vi "play_FXP_AFMss_MPC_DistEst_singleAxis.vi"() -> ()   [LabVIEW 2017]
uses:
  fpga_VIs/fixed-point/single-axis/fxp_mpc/fgm_pipiline/quadProgParams_pipe.ctl
  fpga_VIs/fixed-point/typeDefs/FXPControlParams_distEst.ctl
  <vilib>/Analysis/Matrix/Datatypes/RealMatrix.ctl
  fpga_fp_interface_lib/fpga_interface_types/boolean_indicators.ctl
  controls/ObserverMatrices.ctl
  <vilib>/userdefined/High Color/nirio_resource_hc.ctl
  <vilib>/Utility/error.llb/DialogType.ctl
  <vilib>/Utility/file.llb/Read Delimited Spreadsheet (DBL).vi
  <vilib>/FPGAPlugInAG/cRIO-9082/niLvFpga_Open_cRIO-9082.vi
  <vilib>/rvi/interface/common/dynamic/niFpgaDynamicAddResources.vi
  <vilib>/FPGAPlugInAG/Dynamic/niLvFpga_Reset_Dynamic.vi
  <vilib>/rvi/interface/common/niFpgaWaitOnOcc.vi
  <vilib>/Utility/error.llb/Error Cluster From Error Code.vi
  <vilib>/rvi/errors/niLvFpgaAdjustHostInterfaceError.vi
  <vilib>/FPGAPlugInAG/Dynamic/niLvFpga_Run_Dynamic.vi
  <vilib>/RVI Host/nirviSupport.llb/nirviErrorClusterFromErrorCode.vi
  fpga_fp_interface_lib/write_FP_data_to_fpga.vi
  fpga_fp_interface_lib/acquire_FXP_18-5_FIFO_1.vi
  <vilib>/Analysis/Matrix/Numeric/Conversions/Array To Matrix - RA2.vi
  <vilib>/Utility/file.llb/Write To Spreadsheet File (DBL).vi
  <vilib>/FPGAPlugInAG/Dynamic/niLvFpga_Close_Dynamic.vi
  <vilib>/rvi/interface/nirviOpenFPGA/nirviOpenFPGA.xnode
  FPGA Bitfiles/XYpeizocontrol_FPGATarget_FXPAFMssMPCsingle_axis.lvbitx
  <vilib>/rvi/interface/nirviMethod/nirviMethod.xnode
  <vilib>/rvi/interface/nirviReadWriteControl/nirviReadWriteControl.xnode
  <vilib>/rvi/interface/nirviCloseFPGA/nirviCloseFPGA.xnode
  <vilib>/rvi/errors/niLvFpgaMergeErrorWithErrorCode.vi
  <vilib>/rvi/interface/Simulation/niFpgaSimulationCallBeginRW.vi
  <vilib>/rvi/interface/nirviMethod/StockFPGA_InlinedMethodWaitForSingleIRQ.vi
  <vilib>/FPGAPlugInAG/Dynamic/niLvFpga_WaitOnIrq_Dynamic.vi
  <vilib>/FPGAPlugInAG/Dynamic/niLvFpga_AcknowledgeIrq_Dynamic.vi
  <vilib>/FPGAPlugInAG/Dynamic/niLvFpga_ConfigureFifo_Dynamic.vi
  NiFpgaLv.dll
  <vilib>/Analysis/Matrix/NI_Matrix.lvlib
  <vilib>/FPGAPlugInAG/Dynamic/niLvFpga_WriteFifo_Dynamic.vi
  labview/utils_lib/utils.lvlib
panel:
  out "first row":dbl[](array[numeric])
  out "elements left":i32=1
  in  "N_sat":i32
  in  "wsat_s":T1
  in  "d_s":T1
  in  "N_hyst":i32
  in  "w-s":T1
  in  "r_s":T1
  in  "TF Order":i32
  in  "den":T1
  in  "num":T1
  out "u_k out":fxp<+/-,32,5>
  out "size(s)":i32[](array[numeric])
  in  "Tab Control":T2(tab)
  in  "traj_path":path=path "C:/Users/arnold/Documents/MATLAB/afm_mpc_journal/data/MPCControls01.csv"
  in  "control_data_path":path=path "C:/Users/arnold/Documents/MATLAB/afm_mpc_journal/data/MPCControls01.csv"
  in  "outputDataPath":path=path "Z:/mpc-journal/step-exps/expOut_multiAxis_mpc_tmp.csv"
  in  "dry_run":bool
  out "XY Graph":cluster{dbl[], "2D Data Out":dbl[]}[](graph)
  out "QP_params":T3={"maxIter"=0, "nuN"=24, "Ns_mpc"=0, "-beta"=-0.9987945556640625, "beta+1"=1.9987945556640625}
  out "ControlParams":T4={"umax"=3.0, "Ns_obs/cntrl"=0, "ref_f_VEC"=[0.0, 0.0], "du_max"=0.0}
  in  "TsTicks":i32=1600
  in  "umax":dbl=1.0 format="%#_13g"
  in  "ymax":dbl=4.0 format="%#_13g"
  in  "Iters":i32=25
  in  "SettleTicks":i32=10
  in  "ABORT":bool
  out "Fifo matrix TimeOUt":bool
  in  "ref":dbl=1.0 format="%#_13g"
  out "Loop Ticks (benchmark)":i16
  in  "maxIter":u16=20
  out "boolean  indicators":T5
  out "error out (stage 2)":errorcluster
  out "Error Out (stage 1)":errorcluster
  out "x-x(0)":fxp<+/-,18,5>
  out "ControlMatrices":T6
  out "MPC matrices":dbl[][](array[numeric])
  out "result_data":T1
  out "Empty Elements Remaining":u32
  # "NOTE: Ns is the number of states in the plant. The number of states in the \nobserver is Ns+1. Thus, for B, L, C, and A, we use NS+1. For K and Xss, we use Ns\nbecause the controller does not operate on the disturbance state, Xd."
  # "yk\nulin\ndu\nu_inv\nIpow\nX"
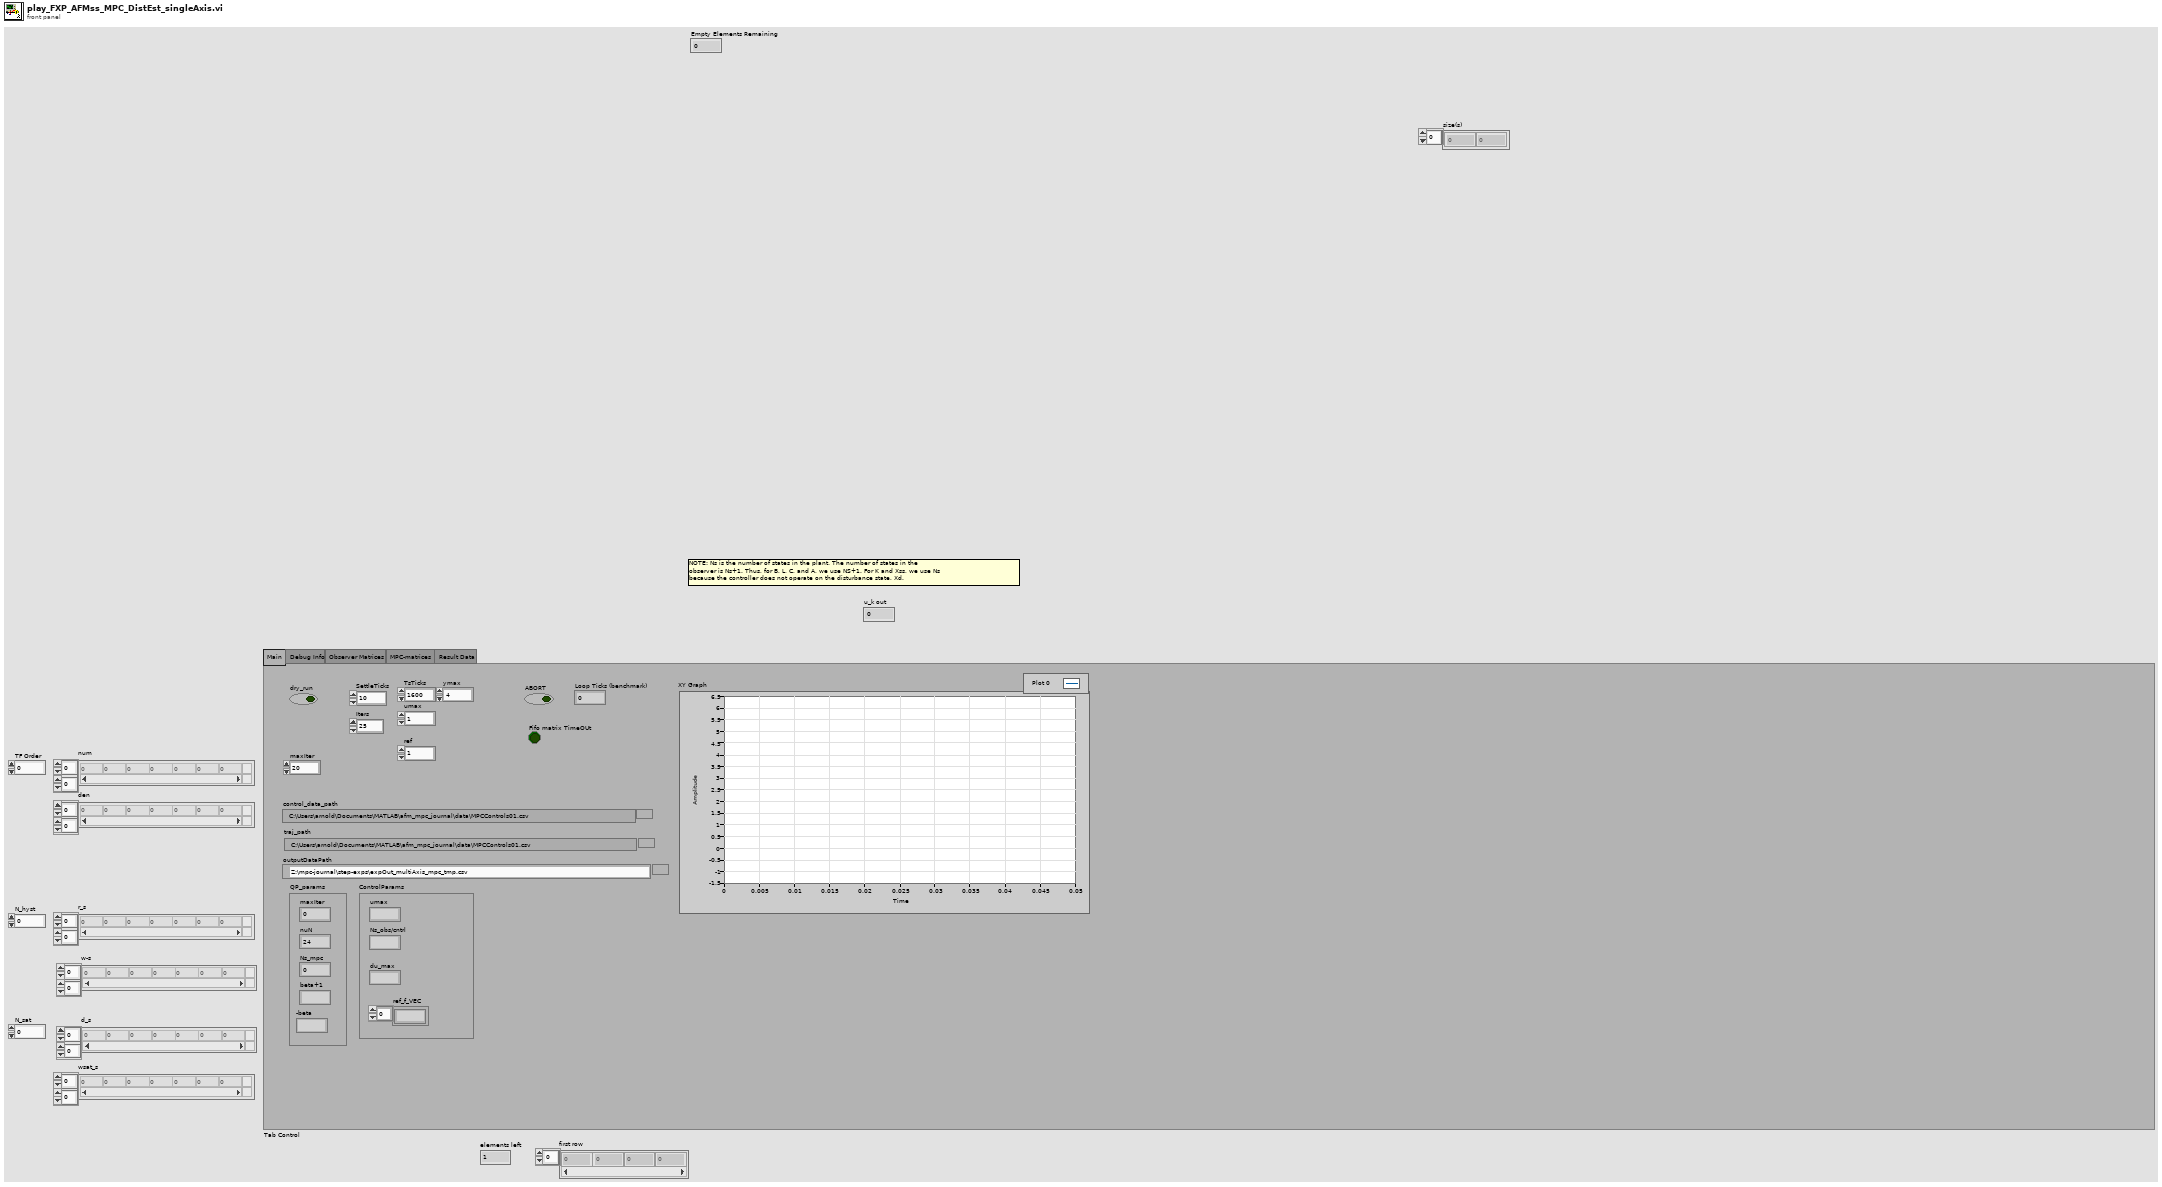
[diagram p1: front panel]
types:
  T1 = typedef "NI_Matrix.lvlib/RealMatrix.ctl" = dbl[][]
  T2 = enum32{"Main", "Debug Info", "Observer Matrices", "MPC-matrices", "Result Data"}
  T3 = typedef "quadProgParams_pipe.ctl" = cluster{"maxIter":u16, "nuN":u16, "Ns_mpc":u16, "-beta":fxp<+/-,18,2>, "beta+1":fxp<+/-,18,2>}
  T4 = typedef "FXPControlParams_distEst.ctl" = cluster{"umax":fxp<+/-,18,5>, "Ns_obs/cntrl":u8, "ref_f_VEC":fxp<+/-,32,5>[], "du_max":fxp<+/-,18,5>}
  T5 = typedef "boolean_indicators.ctl" = cluster{"unstable-z-traj":bool, "input fifo time-out":bool, "logging fifo timeout":bool, "scanning finished":bool, "unstable-x-traj":bool, "unstable-y-traj":bool, "ABORT":bool, "All Measurements Done":bool, "fpga_finished":bool}
  T6 = typedef "ObserverMatrices.ctl" = cluster{"Az":fxp<+/-,32,4>[][], "Bz":dbl[][], "Lz":dbl[][], "Kz":dbl[][], "NxNu":dbl[][]}
  T7 = typedef "nirio_resource_hc.ctl" = tag
  T8 = cluster{"unstable-z-traj":bool, "input fifo time-out":bool, "logging fifo timeout":bool, "scanning finished":bool, "unstable-x-traj":bool, "unstable-y-traj":bool, "ABORT":bool, "All Measurements Done":bool, "fpga_finished":bool}
  T9 = typedef "DialogType.ctl" = u16
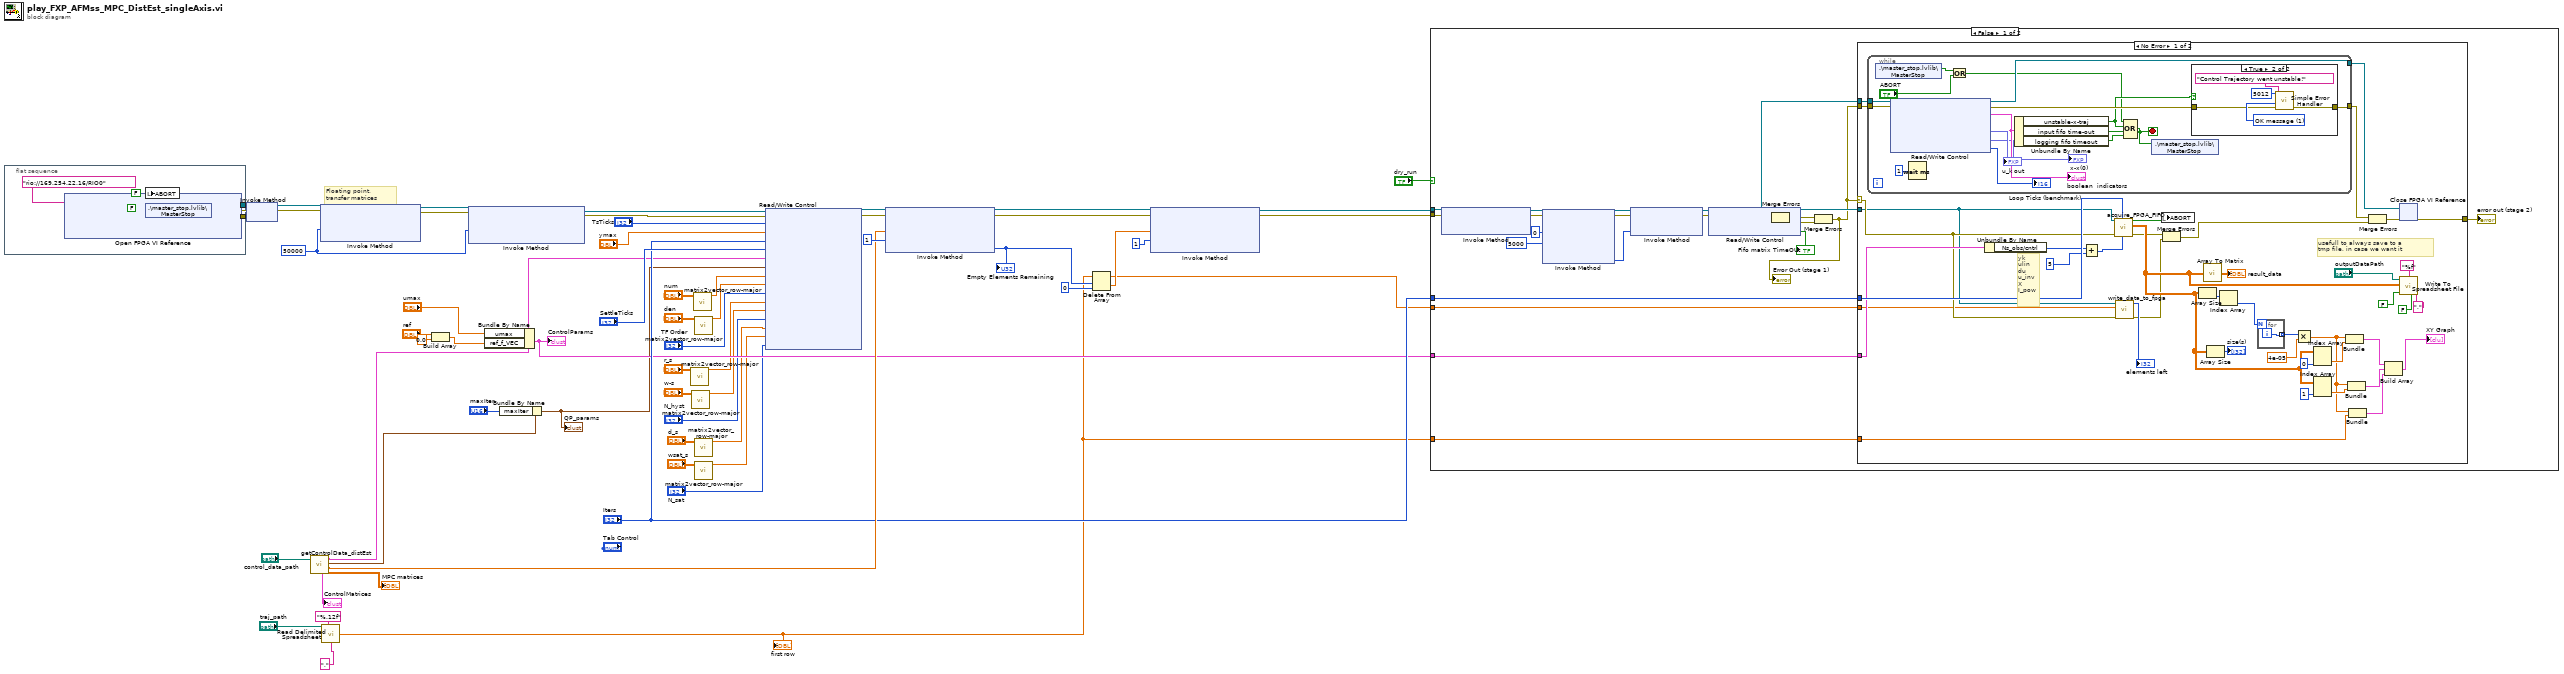
[diagram p0: block diagram]
diagram:
  w38 = u32 50000 ("Requested Depth")
  # "Floating point, \ntransfer matrices"
  n1 = flat-sequence {
    tunnel: [w61] -> w52
    tunnel: [w63] -> w50
    frame #0 {
      n2 = xnode "Open FPGA VI Reference"("resource name"=T7 "rio://169.254.22.16/RIO0") -> ("FPGA VI Reference Out"=w63:refnum<k20>, "error out"=w60:errorcluster)  [unwired: 1 in]
      n3 = shared-variable ".\\master_stop.lvlib\\MasterStop"(FALSE ("MasterStop"), error in=w60) -> (error out=w61:errorcluster)
      n4 = local write "ABORT"(FALSE ("ABORT")) -> ()
    }
  }
  n5 = xnode "Invoke Method"("FPGA VI Reference In"=w50, "error in"=w52) -> ("FPGA VI Reference Out"=w49:refnum<k20>, "error out"=w48:errorcluster)
  n6 = call "getControlData_distEst.vi"("system matricec path"="control_data_path") -> ("MPC matrices"=→"MPC matrices":dbl[][], "AllMatrix"=w42:dbl[], "QP_params"=w31:T3, "ControlParams"=w36:T4, "ControlMatrices"=→"ControlMatrices":T6)  [unwired: 6 in]
  n7 = xnode "Invoke Method"("FPGA VI Reference In"=w49, "error in"=w48, "Requested Depth"=w38) -> ("FPGA VI Reference Out"=w47:refnum<k20>, "error out"=w46:errorcluster)  [unwired: 1 out]
  n8 = call-poly <vilib>:"Read Delimited Spreadsheet.vi"("file path (dialog if empty)"="traj_path", "format (%.3f)"="%.12f", "delimiter (\\t)"="," ("format (%.3f)")) -> ("first row"=w1:dbl[])  [unwired: 7 in, 5 out]
  "first row" <- w1
  n9 = Build Array("ref", 0.0 ("element")) -> (w32:dbl[])
  n10 = xnode "Invoke Method"("FPGA VI Reference In"=w47, "error in"=w46, "Requested Depth"=w38) -> ("FPGA VI Reference Out"=w45:refnum<k20>, "error out"=w44:errorcluster)  [unwired: 1 out]
  n11 = Bundle By Name(cluster=w36, "umax"="umax", "ref_f_VEC"=w32) -> (w35:T4)
  "ControlParams" <- w35
  n12 = Bundle By Name(cluster=w31, "maxIter"="maxIter") -> (w29:T3)
  "QP_params" <- w29
  n13 = call "matrix2vector_row-major.vi"("Matrix"="r_s") -> ("vector"=w21:dbl[])  [unwired: 10 in]
  n14 = call "matrix2vector_row-major.vi"("Matrix"="w-s") -> ("vector"=w20:dbl[])  [unwired: 10 in]
  n15 = call "matrix2vector_row-major.vi"("Matrix"="num") -> ("vector"=w24:dbl[])  [unwired: 10 in]
  n16 = call "matrix2vector_row-major.vi"("Matrix"="den") -> ("vector"=w23:dbl[])  [unwired: 10 in]
  n17 = call "matrix2vector_row-major.vi"("Matrix"="d_s") -> ("vector"=w15:dbl[])  [unwired: 10 in]
  n18 = call "matrix2vector_row-major.vi"("Matrix"="wsat_s") -> ("vector"=w14:dbl[])  [unwired: 10 in]
  n19 = xnode "Read/Write Control"("FPGA VI Reference In"=w45, "error in"=w44, "TsTicks"="TsTicks", "ymax"="ymax", "iters"="Iters", "Settle Ticks"="SettleTicks", "ControlParams_distEst"=w35, "QP_params"=w29, "Num"=w24, "Den"=w23, "TF Order"="TF Order", "r_s"=w21, "w_s"=w20, "N_hyst"="N_hyst", "d_s"=w15, "wsat_s"=w14, "N_sat"="N_sat") -> ("FPGA VI Reference Out"=w55:refnum<k20>, "error out"=w54:errorcluster)
  n20 = xnode "Invoke Method"("FPGA VI Reference In"=w55, "error in"=w54, "Data"=w42, "Timeout (ms)"=1) -> ("FPGA VI Reference Out"=w10:refnum<k20>, "error out"=w9:errorcluster, "Empty Elements Remaining"=w5:u32)
  "Empty Elements Remaining" <- w5
  n21 = Delete From Array(array=w1, length=w5, index=0) -> (deleted portion=w4:dbl[], array with subset deleted=w2:dbl[])
  n22 = xnode "Invoke Method"("FPGA VI Reference In"=w10, "error in"=w9, "Data"=w4, "Timeout (ms)"=1) -> ("FPGA VI Reference Out"=w8:refnum<k20>, "error out"=w7:errorcluster)  [unwired: 1 out]
  n23 = case shown="False" "dry_run" {
    tunnel: w7 -> [w86 _]
    tunnel: "Iters" -> [w74 _]
    tunnel: w35 -> [w72 _]
    tunnel: w8 -> [w67 _]
    tunnel: w2 -> [w65 _]
    tunnel: w1 -> [w66 _]
    frame False {
      n24 = xnode "Invoke Method"("FPGA VI Reference In"=w67, "error in"=w86) -> ("FPGA VI Reference Out"=w77:refnum<k20>, "error out"=w78:errorcluster)  [unwired: 1 in]
      n25 = xnode "Invoke Method"("FPGA VI Reference In"=w77, "error in"=w78, "IRQ Number(s)"=0, "Timeout (ms)"=5000) -> ("FPGA VI Reference Out"=w83:refnum<k20>, "error out"=w84:errorcluster, "IRQ(s) Asserted"=w80:i32)  [unwired: 1 out]
      n26 = xnode "Invoke Method"("FPGA VI Reference In"=w83, "error in"=w84, "IRQ Number(s)"=w80) -> ("FPGA VI Reference Out"=w82:refnum<k20>, "error out"=w81:errorcluster)
      n27 = xnode "Read/Write Control"("FPGA VI Reference In"=w82, "error in"=w81) -> ("FPGA VI Reference Out"=w73:refnum<k20>, "error out"=w85:errorcluster, "Error Out"=w69:errorcluster, "Matrix FIFO  TimeOut"=→"Fifo matrix TimeOUt":bool)
      n28 = Merge Errors(w85, w69) -> (w70:errorcluster)
      n29 = Merge Errors(w70, w69) -> (w68:errorcluster)
      "Error Out (stage 1)" <- w68
      n30 = case shown="No Error" w68 {
        selector: w68 -> [w99 w152]
        tunnel: [w126 w152] -> w75
        tunnel: w73 -> [w125 _]
        tunnel: w68 -> [w124 _]
        tunnel: w74 -> [w121 _]
        tunnel: w73 -> [w98 _]
        tunnel: w72 -> [w101 _]
        tunnel: w66 -> [w92 _]
        tunnel: w65 -> [w90 _]
        frame No Error {
          # "yk\nulin\ndu\nu_inv\nX\nI_pow"
          # "usefull to always save to a \ntmp file, in case we want it"
          n31 = while {
            tunnel: w125 -> [w144]
            tunnel: w124 -> [w143]
            tunnel: [w141] -> w123
            tunnel: [w140] -> w122
            stop <- w139 stop-if-true
            n32 = shared-variable ".\\master_stop.lvlib\\MasterStop"() -> (w134:bool)  [unwired: 1 in, 1 out]
            n33 = xnode "Read/Write Control"("FPGA VI Reference In"=w144, "error in"=w143) -> ("FPGA VI Reference Out"=w140:refnum<k20>, "error out"=w142:errorcluster, "boolean  indicators"=w138:T8, "x-x(0)"=→"x-x(0)":fxp<+/-,18,5>, "u_k"=→"u_k out":fxp<+/-,32,5>, "Loop Ticks (benchmark)"=→"Loop Ticks (benchmark)":i16)  [unwired: 1 out]
            "boolean  indicators" <- w138
            n34 = Wait (ms)(milliseconds to wait=u32 1) -> ()  [unwired: 1 out]
            n35 = Or(x=w134, y="ABORT") -> (x .or. y?=w132:bool)
            n36 = Unbundle By Name(w138) -> ("unstable-x-traj"=w136:bool, "input fifo time-out"=w137:bool, "logging fifo timeout"=w135:bool)
            n37 = Compound Arithmetic op=OR(w132, w136, w137, w135) -> (w139:bool)
            n38 = shared-variable ".\\master_stop.lvlib\\MasterStop"(w139) -> ()  [unwired: 1 in, 1 out]
            n39 = case shown="True" w136 {
              tunnel: w142 -> [w146 w148]
              tunnel: [w146 w147] -> w141
              frame False {
              }
              frame True {
                w151 = T9 1 items=["no dialog", "OK message", "continue or stop message", "OK message + warnings", "continue/stop + warnings"] ("type of dialog (OK msg:1)")
                n40 = call <vilib>:"Simple Error Handler.vi"("error code (no error:0)"=5012, "error source (\" \")"="Control Trajectory went unstable!" ("error source (\" \")"), "type of dialog (OK msg:1)"=w151, "error in (no error)"=w148) -> ("error out"=w147:errorcluster)  [unwired: 1 in, 4 out]
              }
            }
          }
          n41 = Unbundle By Name(w101) -> ("Ns_obs/cntrl"=w87:u8)
          n42 = Add(x=w87, y=u8 5) -> (x+y=w119:u8)
          n43 = call-poly "acquire_FPGA_FIFO.vi"("numChannels"=w119, "Iters"=w121, "error in"=w99, "FPGA Interface"=w98) -> ("error out"=w96:errorcluster, "2D Data Out"=w100:dbl[][], "acquisition done"=w120:bool)  [unwired: 3 in, 2 out]
          n44 = call-poly "write_data_to_fpga.vi"("error in"=w99, "all rows"=w90, "FPGA Interface"=w98) -> ("error out"=w94:errorcluster, "elements left"=→"elements left":i32)  [unwired: 7 in]
          n45 = local write "ABORT"(w120) -> ()
          n46 = Merge Errors(w96, w94) -> (w95:errorcluster)
          n47 = Array Size(array=w100) -> (size(s)=w113:i32[])
          n48 = call-poly <vilib>:"Array To Matrix.vi"("Real 2D Array"=w100) -> ("Real Matrix"=→"result_data":T1)
          n49 = Array Size(array=w100) -> (size(s)=→"size(s)":i32[])
          n50 = Index Array(array=w113) -> (element=w112:i32)  [unwired: 1 in]
          n51 = for {
            N: w112 -> [_]
            tunnel: [w128] -> w111 mode=indexing
            i -> [w128]
          }
          n52 = Multiply(x=w111, y=4e-05) -> (x*y=w93:dbl[])
          n53 = Index Array(array=w100, index (col)=0 ("disabled index (col)")) -> (element=w109:dbl[])  [unwired: 1 in]
          n54 = Index Array(array=w100, index (col)=1 ("index (row)")) -> (element=w108:dbl[])  [unwired: 1 in]
          n55 = Bundle(w93, "2D Data Out"=w109) -> (w106:cluster{dbl[], "2D Data Out":dbl[]})  [unwired: 1 in]
          n56 = Bundle(w93, "2D Data Out"=w108) -> (w107:cluster{dbl[], "2D Data Out":dbl[]})  [unwired: 1 in]
          n57 = Bundle(w93, "first row"=w92) -> (w91:cluster{dbl[], "first row":dbl[]})  [unwired: 1 in]
          n58 = Merge Errors(w123, w95) -> (w127:errorcluster)
          n59 = Build Array(w106, w107, w91) -> (→"XY Graph":cluster{dbl[], "first row":dbl[]}[])
          n60 = xnode "Close FPGA VI Reference"("FPGA VI Reference In"=w122, "error in"=w127) -> ("error out"=w126:errorcluster)
          n61 = call-poly <vilib>:"Write To Spreadsheet File.vi"("delimiter (\\t)"=",", "transpose? (no:F)"=FALSE, "format (%.3f)"="%f", "append to file? (new file:F)"=FALSE, "2D data"=w100, "file path (dialog if empty)"="outputDataPath") -> ()  [unwired: 2 in, 1 out]
        }
        frame Error {
        }
      }
      "error out (stage 2)" <- w75
    }
    frame True {
    }
  }
